vi "LoadImage.vi"(6 "fuLoad":u32(ring)=16 items=["LR_CREATEDIBSECTION"=8192, "LR_DEFAULTCOLOR"=0, "LR_DEFAULTSIZE"=64, "LR_LOADFROMFILE"=16, "LR_LOADMAP3DCOLORS"=4096, "LR_LOADTRANSPARENT"=32, "LR_MONOCHROME"=1, "LR_SHARED"=32768, "LR_VGACOLOR"=128], 8 "error in (no error)":errorcluster, 9 "size":cluster{"cx":i32, "cy":i32}={"cx"=32, "cy"=32}, 10 "type":u32(ring) items=["IMAGE_BITMAP", "IMAGE_CURSOR", "IMAGE_ICON"], 11 "name":string) -> (0 "error out":errorcluster, 3 "HANDLE":u32)   [LabVIEW 2019]
uses:
  user32.dll
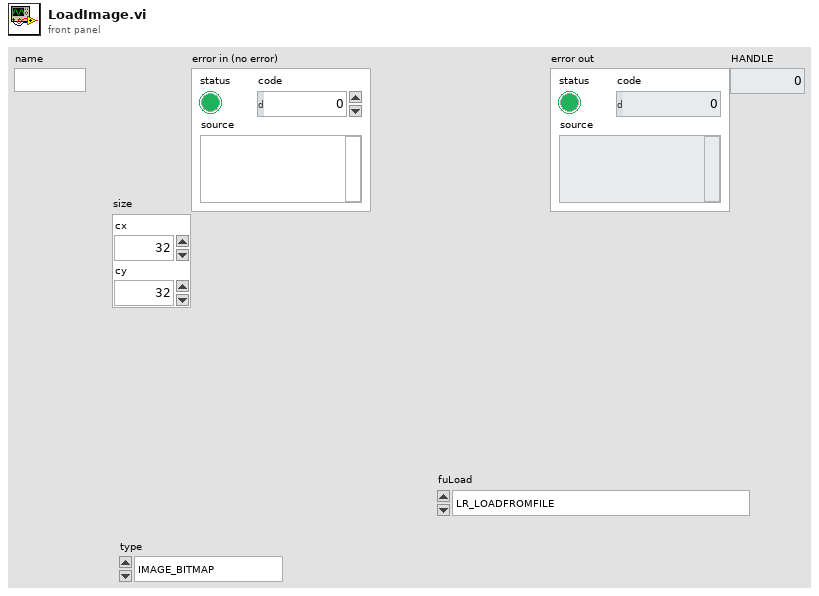
[diagram p1: front panel]
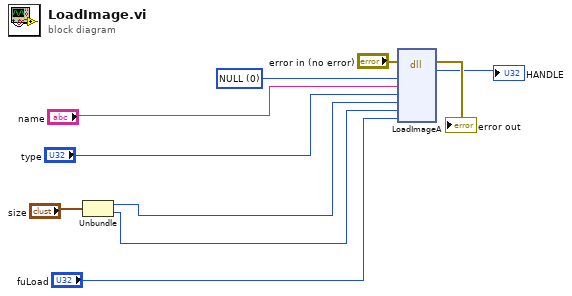
[diagram p0: block diagram]
diagram:
  w10 = 0 items=["NULL"]
  n1 = Unbundle("size") -> ("cx"=w6:i32, "cy"=w5:i32)
  n2 = dll-call lib="user32.dll" fn="LoadImageA"(error in="error in (no error)", "hInst"=w10, "name"="name", "type"="type", "cx"=w6, "cy"=w5, "fuLoad"="fuLoad") -> (error out=→"error out":errorcluster, "HANDLE"=→"HANDLE":u32)  [unwired: 8 in, 1 out]
